vi "svc_Convert Spectrum Cluster to XY Cluster.vi"(4 "spectrum cluster":cluster{"x0":dbl, "dx":dbl, "Y":dbl[]}={"x0"=0.0, "dx"=1.0, "Y"=[]}) -> (1 "XY cluster":cluster{"X":dbl[], "Y":dbl[]})   [LabVIEW 2017]
doc: "Converts an evenly spaced spectrum of the form {x0 dx [Y]} to XY data of the form {[X] [Y]}."
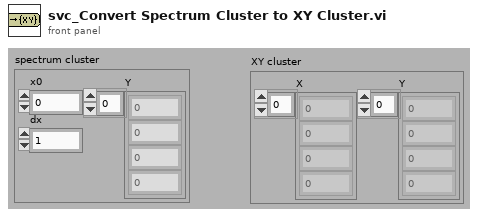
[diagram p1: front panel]
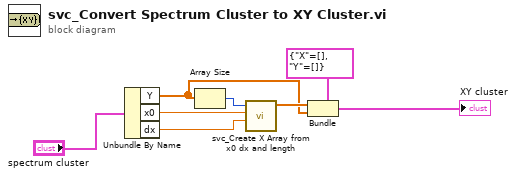
[diagram p0: block diagram]
diagram:
  n1 = Unbundle By Name("spectrum cluster") -> ("Y"=w5:dbl[], "x0"=w3:dbl, "dx"=w1:dbl)
  n2 = Array Size(array=w5) -> (size(s)=w2:i32)
  n3 = call <vilib>:"svc_Create X Array from x0 dx and length.vi"("dx"=w1, "x0"=w3, "length"=w2) -> ("X"=w6:dbl[])  [unwired: 8 in]
  n4 = Bundle(cluster=cluster{"X":dbl[], "Y":dbl[]} {"X"=[], "Y"=[]}, "X"=w6, "Y"=w5) -> (→"XY cluster":cluster{"X":dbl[], "Y":dbl[]})
